vi "getXMLTestExtension.vi"(9 "indent level":i32, 10 "testcases":T1[](array[typedef])) -> (2 "XML testcases":string[](array[string]))   [LabVIEW 2013]
uses:
  Test Report/Test Report.lvclass
  Test Report.JUnit.lvclass
  testcase -- cluster.ctl
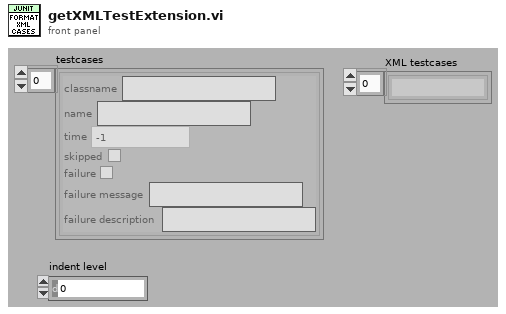
[diagram p1: front panel]
types:
  T1 = typedef "Caraya.lvlib/Test Report.JUnit.lvclass/testcase -- cluster.ctl" = cluster{"classname":string, "name":string, "time":dbl, "skipped":bool, "failure":bool, "failure message":string, "failure description":string}
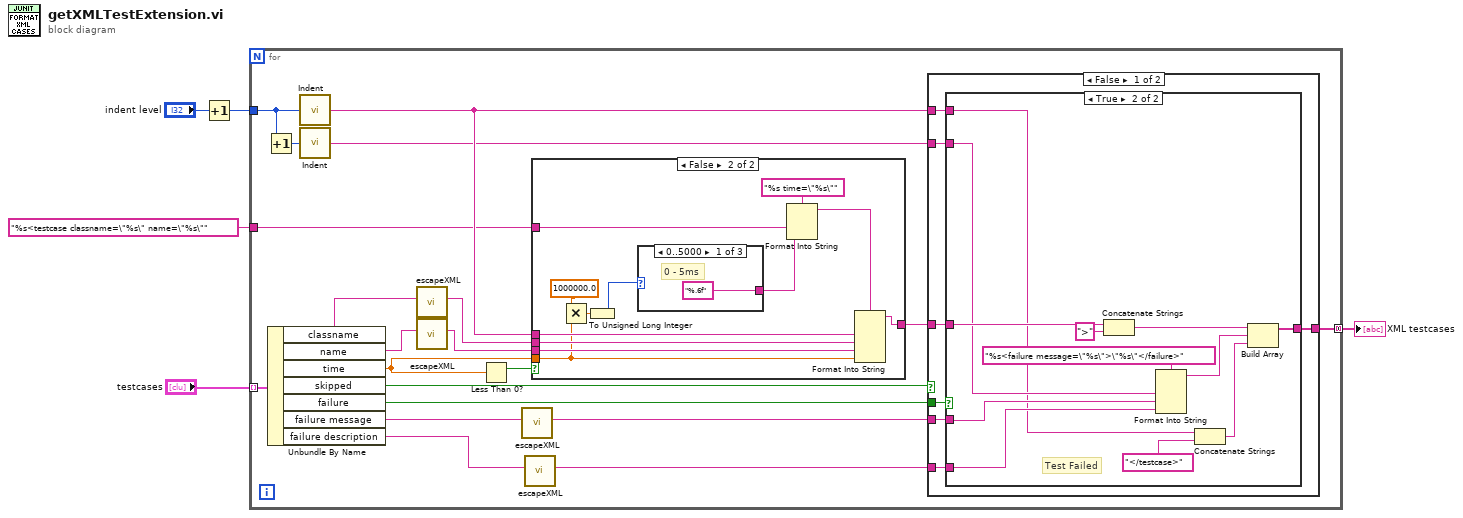
[diagram p0: block diagram]
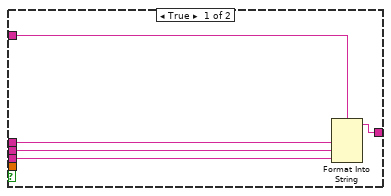
[diagram p2: hidden frame]
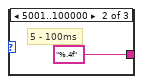
[diagram p3: hidden frame]
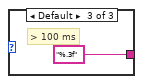
[diagram p4: hidden frame]
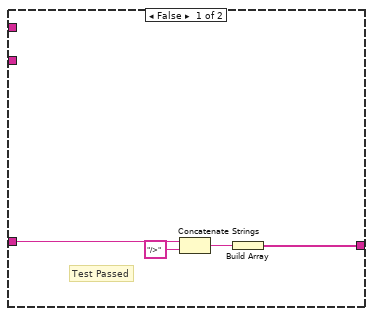
[diagram p5: hidden frame]
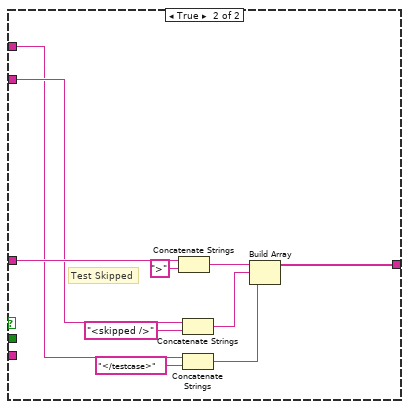
[diagram p6: hidden frame]
diagram:
  n1 = Increment(x="indent level") -> (x+1=w3:i32)
  n2 = for {
    tunnel: "testcases" -> [w25] mode=indexing
    tunnel: w3 -> [w21]
    tunnel: [w17] -> w2 mode=concatenating
    tunnel: "%s<testcase classname=\"%s\" name=\"%s\"" -> [w14]
    n3 = Increment(x=w21) -> (x+1=w19:i32)
    n4 = Unbundle By Name(w25) -> ("classname"=w13:string, "name"=w11:string, "time"=w16:dbl, "skipped"=w24:bool, "failure"=w23:bool, "failure message"=w9:string, "failure description"=w7:string)
    n5 = call "Indent.vi"("Numeric"=w21) -> ("string"=w20:string)
    n6 = call "Indent.vi"("Numeric"=w19) -> ("string"=w18:string)
    n7 = call "escapeXML.vi"("Input String"=w13) -> ("XML-escaped String"=w12:string)  [unwired: 10 in]
    n8 = call "escapeXML.vi"("Input String"=w11) -> ("XML-escaped String"=w10:string)  [unwired: 10 in]
    n9 = Less Than 0?(x=w16) -> (x < 0?=w15:bool)
    n10 = call "escapeXML.vi"("Input String"=w9) -> ("XML-escaped String"=w8:string)  [unwired: 10 in]
    n11 = call "escapeXML.vi"("Input String"=w7) -> ("XML-escaped String"=w6:string)  [unwired: 10 in]
    n12 = case shown="False" w15 {
      tunnel: w10 -> [w30 w42]
      tunnel: w12 -> [w29 w41]
      tunnel: [w28 w40] -> w22
      tunnel: w20 -> [w27 w39]
      tunnel: w16 -> [_ w33]
      tunnel: w14 -> [w26 w38]
      frame True {
        n13 = Format Into String(format string=w26, w27, w29, w30) -> (resulting string=w28:string)  [unwired: 2 in, 1 out]
      }
      frame False {
        n14 = Multiply(x=1000000.0 ("y"), y=w33) -> (x*y=w35:dbl)
        n15 = To Unsigned Long Integer(number=w35) -> (unsigned 32bit integer=w32:u32)
        n16 = case shown="0..5000" w32 {
          tunnel: ["%.6f" "%.4f" "%.3f"] -> w31
          frame 0..5000 {
            # "0 - 5ms"
          }
          frame 5001..100000 {
            # "5 - 100ms"
          }
          frame Default {
            # "> 100 ms"
          }
        }
        n17 = Format Into String(format string="%s time=\"%s\"", w38, w31) -> (resulting string=w36:string)  [unwired: 2 in, 1 out]
        n18 = Format Into String(format string=w36, w39, w41, w42, w33) -> (resulting string=w40:string)  [unwired: 2 in, 1 out]
      }
    }
    n19 = case shown="False" w24 {
      tunnel: [w51 w78] -> w17
      tunnel: w23 -> [w52 _]
      tunnel: w8 -> [w50 _]
      tunnel: w6 -> [w49 _]
      tunnel: w22 -> [w48 w76]
      tunnel: w18 -> [w47 w70]
      tunnel: w20 -> [w46 w69]
      frame False {
        n20 = case shown="True" w52 {
          tunnel: [w53 w61] -> w51
          tunnel: w50 -> [_ w66]
          tunnel: w49 -> [_ w65]
          tunnel: w48 -> [w55 w64]
          tunnel: w47 -> [_ w60]
          tunnel: w46 -> [_ w59]
          frame False {
            # "Test Passed"
            n21 = Concatenate Strings(w55, "/>" ("string")) -> (w54:string)
            n22 = Build Array(w54) -> (w53:string[])
          }
          frame True {
            # "Test Failed"
            n23 = Concatenate Strings(w64, ">" ("string")) -> (w62:string)
            n24 = Format Into String(format string="%s<failure message=\"%s\">\"%s\"</failure>", w60, w66, w65) -> (resulting string=w68:string)  [unwired: 2 in, 1 out]
            n25 = Concatenate Strings(w59, "</testcase>") -> (w57:string)
            n26 = Build Array(w62, w68, w57) -> (w61:string[])
          }
        }
      }
      frame True {
        # "Test Skipped"
        n27 = Concatenate Strings(w76, ">" ("string")) -> (w75:string)
        n28 = Concatenate Strings(w70, "<skipped />") -> (w71:string)
        n29 = Concatenate Strings(w69, "</testcase>") -> (w73:string)
        n30 = Build Array(w75, w71, w73) -> (w78:string[])
      }
    }
  }
  "XML testcases" <- w2
